vi "Add Round Qualified Details.vi"(0 "Qualified for round":string, 1 "Search Element":string, 2 "Event Number":dbl, 4 "file path (dialog if empty)":path=path "E:/Daily Lessons/My Experiments and Results/Elcom Dias/Test2.csv") -> (3 "Match Found":bool)   [LabVIEW 2014]
uses:
  <vilib>/Utility/file.llb/Read From Spreadsheet File (string).vi
  <vilib>/Utility/file.llb/Write To Spreadsheet File (string).vi
panel:
  out "all rows 2":string[][](array[string])
  out "output array 2":string[][](array[string])
  out "output array":string[][](array[string])
  out "j":i32
  out "i":i32
  out "all rows":string[][](array[string])
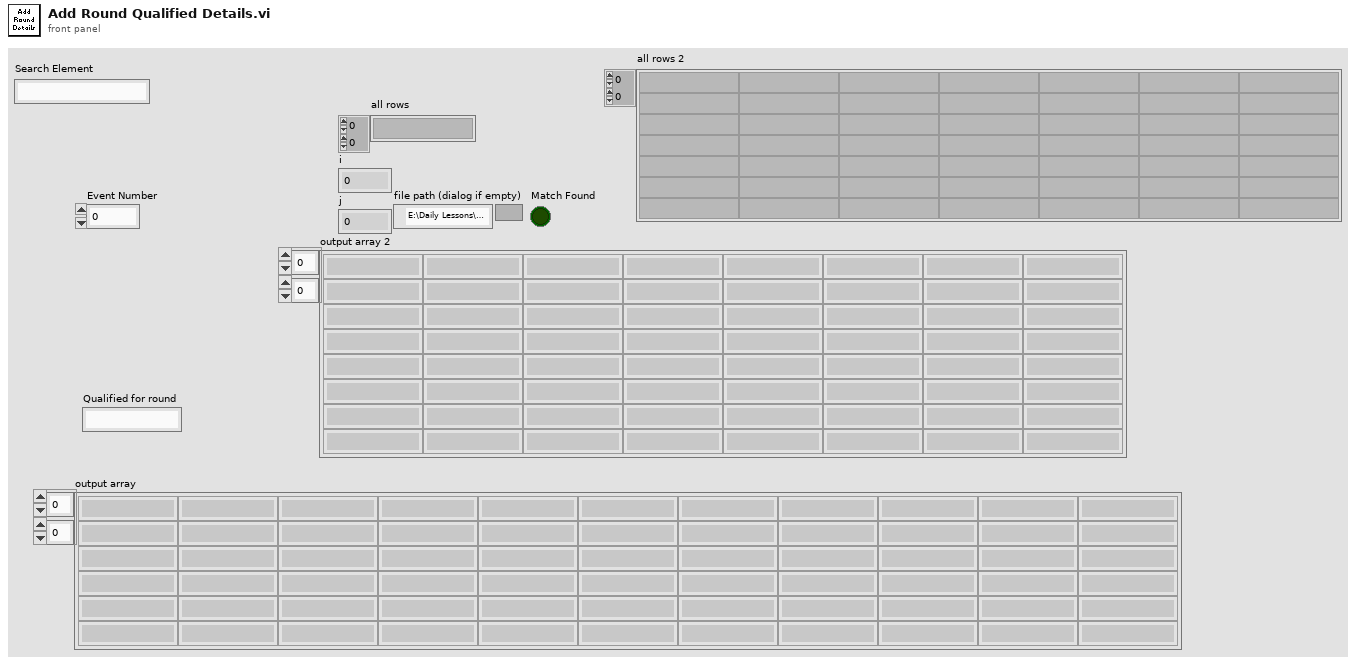
[diagram p1: front panel]
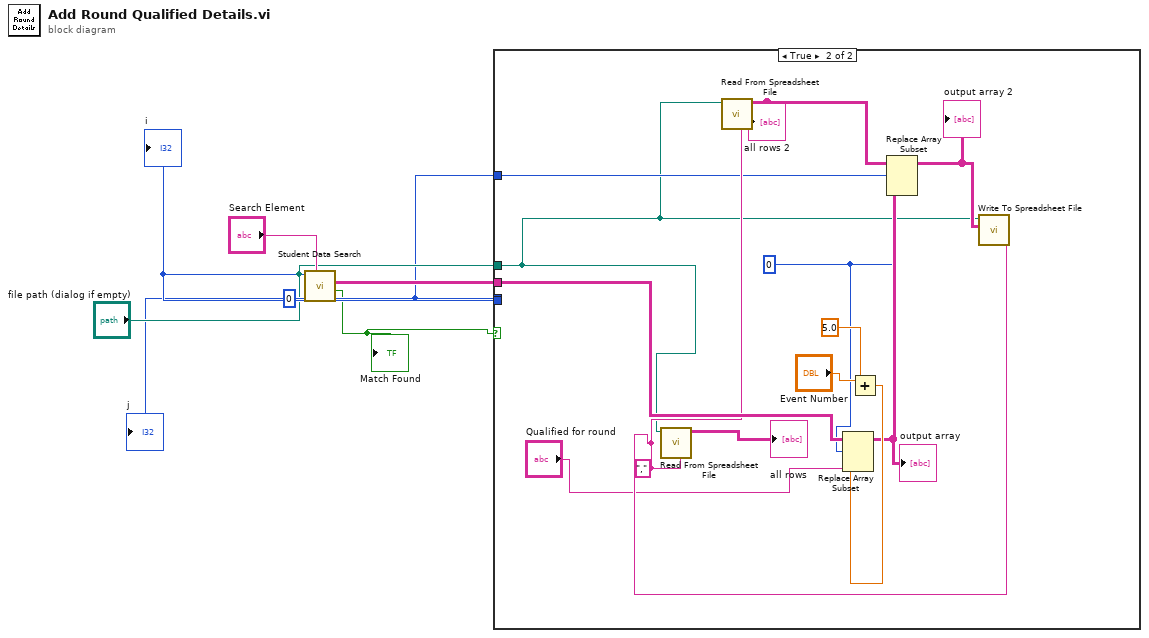
[diagram p0: block diagram]
diagram:
  n1 = call "Student Data Search.vi"("Search Element"="Search Element", "Search Item"=i8 0, "file path (dialog if empty)"="file path (dialog if empty)") -> ("j"=w2:i32, "Match Found"=w1:bool, "subarray"=w5:string[][], "i"=w4:i32)  [unwired: 2 out]
  "i" <- w4
  "j" <- w2
  "Match Found" <- w1
  n2 = case shown="True" w1 {
    tunnel: w5 -> [_ w19]
    tunnel: w2 -> [_ _]
    tunnel: w4 -> [_ _]
    tunnel: "file path (dialog if empty)" -> [_ w9]
    tunnel: w2 -> [_ w10]
    frame False {
    }
    frame True {
      w11 = 0 ("disabled index (col)")
      w12 = "," ("delimiter (\\t)")
      n3 = call-poly <vilib>:"Read From Spreadsheet File.vi"("delimiter (\\t)"=w12, "file path (dialog if empty)"=w9) -> ("all rows"=→"all rows":string[][])  [unwired: 5 in, 4 out]
      n4 = call-poly <vilib>:"Read From Spreadsheet File.vi"("delimiter (\\t)"=w12, "file path (dialog if empty)"=w9) -> ("all rows"=w15:string[][])  [unwired: 5 in, 4 out]
      "all rows 2" <- w15
      n5 = Add(x="Event Number", y=5.0) -> (x+y=w16:dbl)
      n6 = Replace Array Subset(array=w19, new element="Qualified for round", index (row)=w11, index (col)=w16) -> (w14:string[][])
      "output array" <- w14
      n7 = Replace Array Subset(array=w15, new element=w14, index (row)=w10, index (col)=w11) -> (w13:string[][])
      "output array 2" <- w13
      n8 = call-poly <vilib>:"Write To Spreadsheet File.vi"("delimiter (\\t)"=w12, "2D data"=w13, "file path (dialog if empty)"=w9) -> ()  [unwired: 5 in, 1 out]
    }
  }
